vi "Close_Instr.vi"(8 "error in (no error)":errorcluster caption="entrée d'erreur (pas d'erreur)", 11 "Class DIO en entrée":refnum<class "Class Instrument Ana.lvclass">) -> (0 "error out":errorcluster caption="sortie d'erreur", 3 "Class DIO en Sortie":refnum<class "Class Instrument Ana.lvclass">)   [LabVIEW 2020, in "Library Instrument & Equipement.lvlib" / "Library Instruments.lvlib" / "Class Instrument Ana.lvclass"]
uses:
  Class Instrument Ana.lvclass
  Class Instrument Ana.lvclass/Class Instrument Ana.ctl
  Ana/Class Ana (Default)/Class Ana (Default).lvclass
  Instrument (Default)/Class Instrument (Default).lvclass
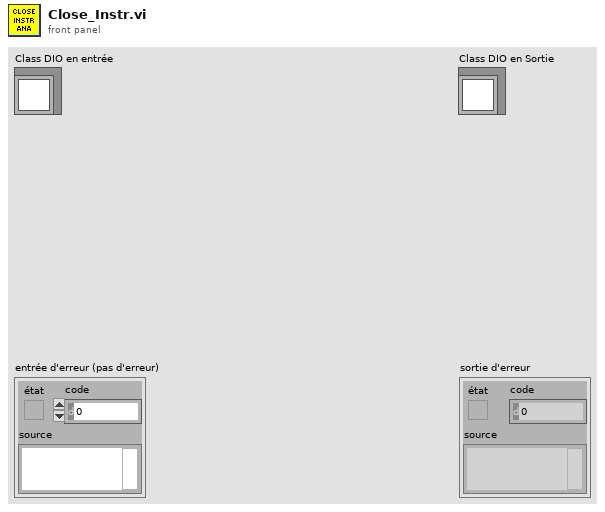
[diagram p1: front panel]
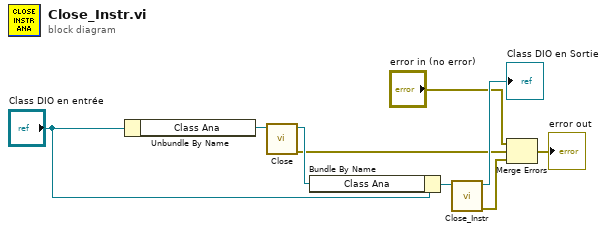
[diagram p0: block diagram]
diagram:
  n1 = Unbundle By Name("Class DIO en entrée") -> ("Class Ana"=w3:refnum<class "Class Ana (Default).lvclass">)
  n2 = call-dynamic "Close.vi"("Class DIO (Default) en entrée"=w3) -> ("error out"=w1:errorcluster, "Class DIO (Default) en sortie"=w2:refnum<class "Class Ana (Default).lvclass">)  [unwired: 9 in]
  n3 = Bundle By Name(cluster="Class DIO en entrée", "Class Ana"=w2) -> (w7:refnum<class "Class Instrument Ana.lvclass">)
  n4 = call-parent "Close_Instr.vi"("Class Instrument (Default) en entrée"=w7) -> ("error out"=w5:errorcluster, "Class Instrument (Default) en sortie"=→"Class DIO en Sortie":refnum<class "Class Instrument Ana.lvclass">)  [unwired: 9 in]
  n5 = Merge Errors("error in (no error)", w1, w5) -> (→"error out":errorcluster)
